vi "Step Builder.vi"(8 "error in (no error)":errorcluster, 11 "Standard Sequence":string[](array[string])) -> (0 "error out":errorcluster, 3 "Step Config out":refnum<class "Step Config.lvclass">)   [LabVIEW 2015, in "Step Config.lvclass"]
uses:
  Step Config.lvclass
  basic steps/Wait Step/Config/Wait Step Config.lvclass
  basic steps/Parallel Step/Config/Parallel Step Config.lvclass
  basic steps/Counter/Config/Counter Config.lvclass
  basic steps/Conditional Jump Step/Config/Conditional Jump Step Config.lvclass
  basic steps/Wait On Boolean/Config/Wait On Boolean Step Config.lvclass
  basic steps/Update Tag Step/Config/Update Tag Configuration/Update Tag Config.lvclass
  basic steps/String Compare/Config/String Compare Config.lvclass
  basic steps/Numeric Limit Compare/Config/Numeric Limit Compare Config.lvclass
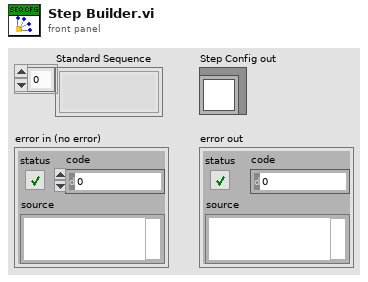
[diagram p1: front panel]
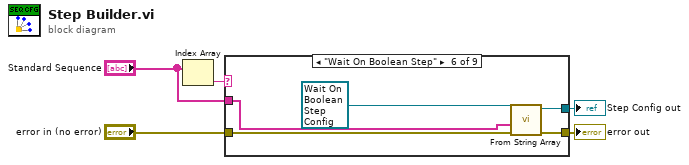
[diagram p0: block diagram]
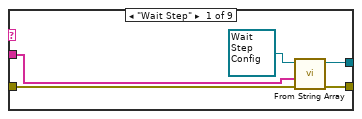
[diagram p2: hidden frame]
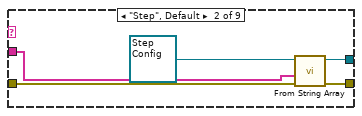
[diagram p3: hidden frame]
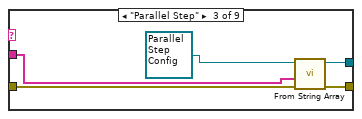
[diagram p4: hidden frame]
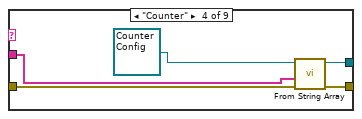
[diagram p5: hidden frame]
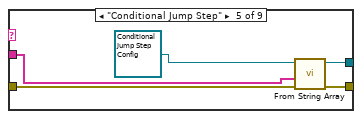
[diagram p6: hidden frame]
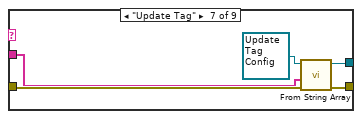
[diagram p7: hidden frame]
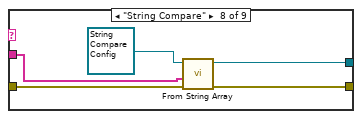
[diagram p8: hidden frame]
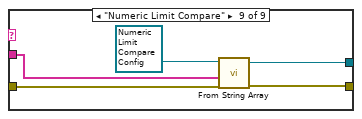
[diagram p9: hidden frame]
diagram:
  n1 = Index Array(array="Standard Sequence") -> (element=w1:string)  [unwired: 1 in]
  n2 = case shown="\"Wait On Boolean Step\"" w1 {
    tunnel: "Standard Sequence" -> [w8 w14 w19 w24 w29 w34 w36 w45 w50]
    tunnel: [w9 w15 w20 w25 w30 w35 w39 w42 w47] -> w3
    tunnel: "error in (no error)" -> [w7 w13 w18 w23 w28 w33 w37 w41 w49]
    tunnel: [w6 w12 w17 w22 w27 w32 w38 w43 w48] -> w5
    frame "Wait Step" {
      n3 = call-dynamic "From String Array.vi"("error in (no error)"=w7, "String Array"=w8, "Wait Step Config in"=refnum<class "Wait Step Config.lvclass"> refnum ("Wait Step Config.lvclass")) -> ("error out"=w6:errorcluster, "Wait Step Config out"=w9:refnum<class "Wait Step Config.lvclass">)  [unwired: 5 in, 2 out]
    }
    frame "Step", Default {
      n4 = call-dynamic "From String Array.vi"("error in (no error)"=w13, "String Array"=w14, "Step Config in"=refnum<class "Step Config.lvclass"> refnum ("Step Config.lvclass")) -> ("error out"=w12:errorcluster, "Step Config out"=w15:refnum<class "Step Config.lvclass">)  [unwired: 5 in, 2 out]
    }
    frame "Parallel Step" {
      n5 = call-dynamic "From String Array.vi"("error in (no error)"=w18, "String Array"=w19, "Parallel Step Config in"=refnum<class "Parallel Step Config.lvclass"> refnum ("Parallel Step Config.lvclass")) -> ("error out"=w17:errorcluster, "Parallel Step Config out"=w20:refnum<class "Parallel Step Config.lvclass">)  [unwired: 5 in, 2 out]
    }
    frame "Counter" {
      n6 = call-dynamic "From String Array.vi"("error in (no error)"=w23, "String Array"=w24, "Counter Config in"=refnum<class "Counter Config.lvclass"> refnum ("Counter Config.lvclass")) -> ("error out"=w22:errorcluster, "Counter Config out"=w25:refnum<class "Counter Config.lvclass">)  [unwired: 5 in, 2 out]
    }
    frame "Conditional Jump Step" {
      n7 = call-dynamic "From String Array.vi"("error in (no error)"=w28, "String Array"=w29, "Conditional Jump Step Config in"=refnum<class "Conditional Jump Step Config.lvclass"> refnum ("Conditional Jump Step Config.lvclass")) -> ("error out"=w27:errorcluster, "Conditional Jump Step Config out"=w30:refnum<class "Conditional Jump Step Config.lvclass">)  [unwired: 5 in, 2 out]
    }
    frame "Wait On Boolean Step" {
      n8 = call-dynamic "From String Array.vi"("error in (no error)"=w33, "String Array"=w34, "Wait On Boolean Config in"=refnum<class "Wait On Boolean Step Config.lvclass"> refnum ("Wait On Boolean Step Config.lvclass")) -> ("error out"=w32:errorcluster, "Wait On Boolean Config out"=w35:refnum<class "Wait On Boolean Step Config.lvclass">)  [unwired: 5 in, 2 out]
    }
    frame "Update Tag" {
      n9 = call-dynamic "From String Array.vi"("error in (no error)"=w37, "String Array"=w36, "Update Tag Config in"=refnum<class "Update Tag Config.lvclass"> refnum ("Update Tag Config.lvclass")) -> ("error out"=w38:errorcluster, "Update Tag Config out"=w39:refnum<class "Update Tag Config.lvclass">)  [unwired: 5 in, 2 out]
    }
    frame "String Compare" {
      n10 = call-dynamic "From String Array.vi"("error in (no error)"=w41, "String Array"=w45, "String Compare Config in"=refnum<class "String Compare Config.lvclass"> refnum ("String Compare Config.lvclass")) -> ("error out"=w43:errorcluster, "String Compare Config out"=w42:refnum<class "String Compare Config.lvclass">)  [unwired: 5 in, 2 out]
    }
    frame "Numeric Limit Compare" {
      n11 = call-dynamic "From String Array.vi"("error in (no error)"=w49, "String Array"=w50, "Numeric Limit Compare Config in"=refnum<class "Numeric Limit Compare Config.lvclass"> refnum ("Numeric Limit Compare Config.lvclass")) -> ("error out"=w48:errorcluster, "Numeric Limit Compare Config out"=w47:refnum<class "Numeric Limit Compare Config.lvclass">)  [unwired: 5 in, 2 out]
    }
  }
  "error out" <- w5
  "Step Config out" <- w3
